vi "CameraSerialController_v04.vi"() -> (4 "图像时间戳":u32=16532020 format="%_32g")   [LabVIEW 2015]
uses:
  <vilib>/Instr/_visa.llb/VISA Configure Serial Port (Instr).vi
  MVCAMSDK.dll
  <vilib>/Analysis/NI_AALBase.lvlib
panel:
  out "连接的字符串":string
  out "转动信号曲线":cluster{"Locations":dbl[], "Amplitudes":dbl[]}[](graph)=[{"Locations"=array[750 elements], "Amplitudes"=array[749 elements]}, {"Locations"=[104.38621227921368, 258.3247060234782, 410.71523318402836, 562.6858730022967, 712.7065754646931], "Amplitudes"=[11153.698204083417, 10559.387052180104, 10974.865031894917, 10500.852817232146, 11059.763900010517]}, {"Locations"=[26.787398227992274, 182.39455189327623, 333.5517219531509, 488.1851999460032, 636.5270621135614], "Amplitudes"=[3284.809720018355, 2039.4564261182056, 3638.2587716464914, 3082.2730888167225, 4217.856016996603]}]
  in  "平移回退":T1=TRUE
  in  "转动回退":T1=TRUE
  in  "转动计数":u16
  in  "转动一次脉冲数":u16=20
  in  "转动前进":T1=TRUE
  in  "平移一次脉冲数":u16=20
  in  "平移计数":u16
  out "variance 2":dbl caption="方差" format="%0.2f"
  in  "flow control (0:none)":u16(ring) caption="流控制（0:无）" items=["无", "XON/XOFF", "RTS/CTS", "XON/XOFF & RTS/CTS", "DTR/DSR", "XON/XOFF & DTR/DSR"]
  in  "stop bits (10: 1 bit)":u16=10 caption="停止位（10: 1位）"
  in  "奇偶 (0:none)":enum16{"None", "Odd", "Even", "Mark", "Space"}(ring) caption="奇偶（0:无）"
  in  "数据比特(默认8)":u16(ring)=8 items=["5"=5, "6"=6, "7"=7, "8"=8]
  in  "波特率(默认9600)":u32=9600
  in  "端口":refnum<visa-resource-name>="COM1"
  in  "平移前进":T1=TRUE
  out "泰伯距离数值":dbl[](array[numeric])=[15.393849374426454, 15.239052716055017, 15.197063981826837, 15.002070246239633]
  out "Locations":dbl[](array[numeric])=[10.438621227921368, 25.832470602347822, 41.07152331840284, 56.268587300229676, 71.27065754646931] caption="上面图像曲线波峰位置"
  out "平移信号曲线":cluster{"Locations":dbl[], "Amplitudes":dbl[]}[](graph)=[{"Locations"=array[750 elements], "Amplitudes"=array[749 elements]}, {"Locations"=[104.38621227921368, 258.3247060234782, 410.71523318402836, 562.6858730022967, 712.7065754646931], "Amplitudes"=[11153.698204083417, 10559.387052180104, 10974.865031894917, 10500.852817232146, 11059.763900010517]}, {"Locations"=[26.787398227992274, 182.39455189327623, 333.5517219531509, 488.1851999460032, 636.5270621135614], "Amplitudes"=[3284.809720018355, 2039.4564261182056, 3638.2587716464914, 3082.2730888167225, 4217.856016996603]}]
  out "光强图 2":dbl[](graph)
  out "variance":dbl caption="方差" format="%0.2f"
  out "相机图像":T2(plugin-control)
  out "横向中心像素光强图":dbl[](graph)
  in  "自定义分辨率设置":bool
  in  "ROI分辨率":T3
  in  "预设分辨率设置":bool
  in  "预设分辨率":T4(radio)
  out "帧速":u32
  out "帧间耗时\n单位：（0.1ms）":u32
  in  "相机枚举":T5(ring)
  in  "自动曝光模式":bool=TRUE caption="软触发"
  in  "手动曝光模式":bool caption="软触发"
  in  "曝光时间，单位微秒":dbl=11000.0 format="%#_6f"
  in  "硬触发模式":bool caption="软触发"
  in  "软触发模式":bool caption="软触发"
  in  "连续模式":bool caption="软触发"
  in  "软触发一帧":bool caption="软触发"
  in  "读取自定义数据":bool
  out "从相机中读出的字符串(32字节)":string
  in  "写入自定义数据":bool
  in  "要写入相机的字符串(32字节)":string
  in  "拍照":bool
  in  "相机参数":bool=TRUE
  in  "Stop":bool
  in  "激活预览":bool=TRUE
  out "Image":T2(plugin-control)
  # "相机原生分辨率设置"
  # "写入自定义数据"
  # "触发设置"
  # "曝光设置"
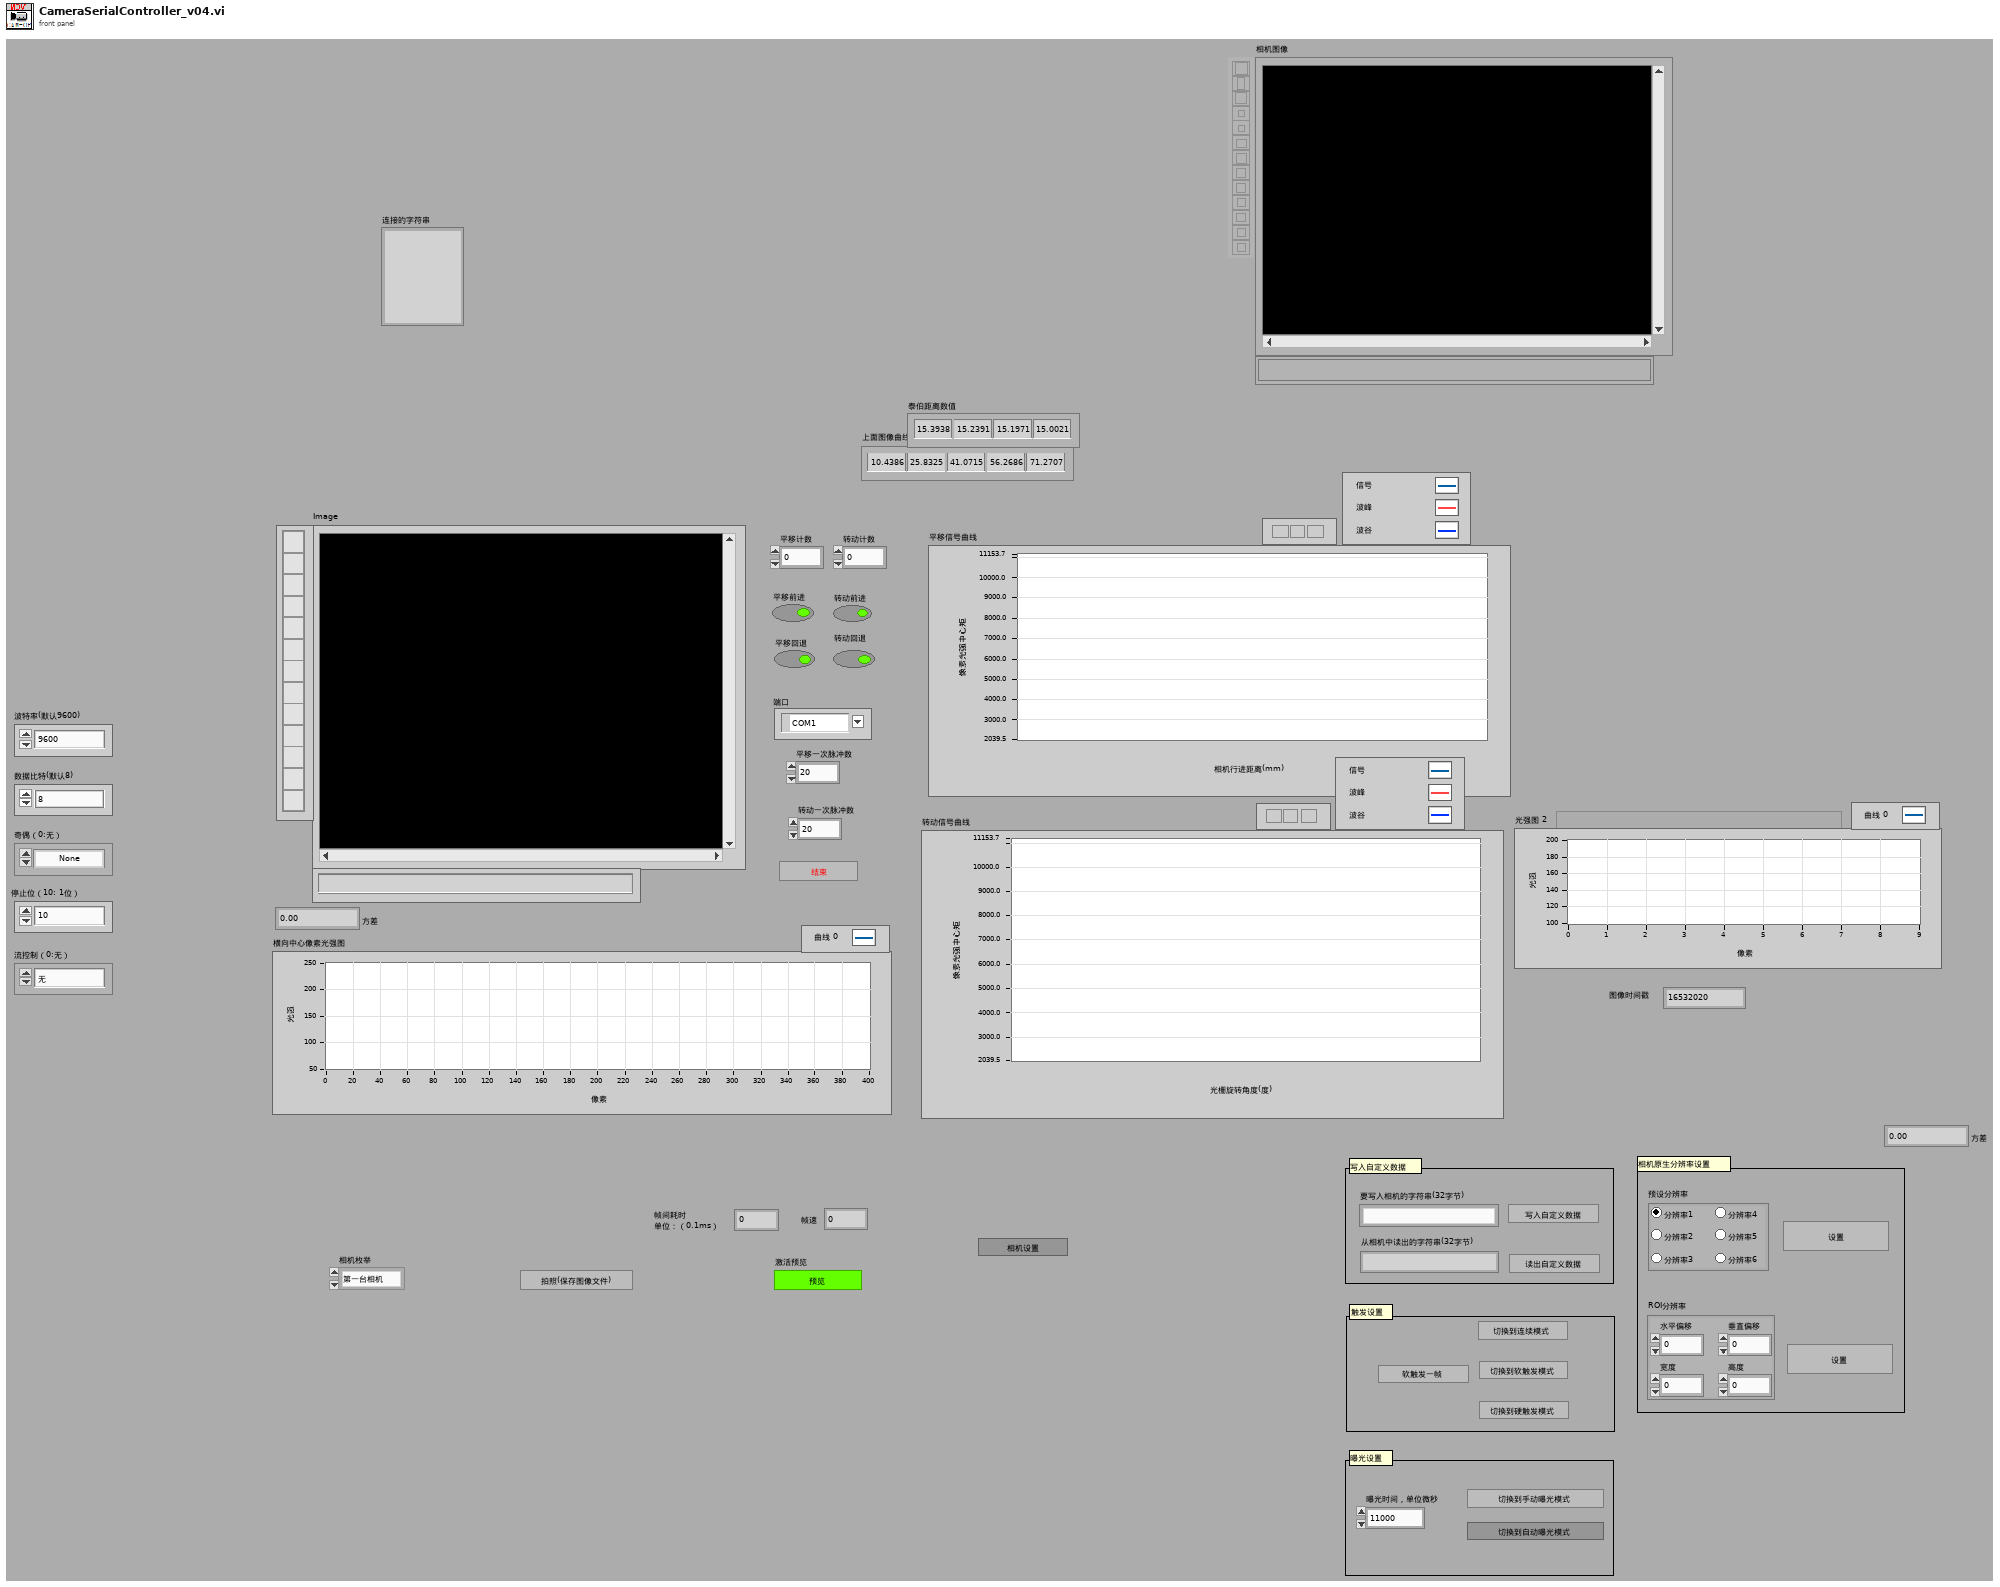
[diagram p1: front panel]
types:
  T1 = typedef "控件 1.ctl" = bool
  T2 = typedef "IMAQ Image.ctl" = refnum<image>
  T3 = cluster{"水平偏移":dbl, "垂直偏移":dbl, "宽度":dbl, "高度":dbl}
  T4 = enum32{"分辨率1", "分辨率2", "分辨率3", "分辨率4", "分辨率5", "分辨率6"}
  T5 = enum16{"第一台相机", "第二台相机", "第三台相机", "第四台相机", "第五台相机"}
  T6 = typedef "Image Type" = u32
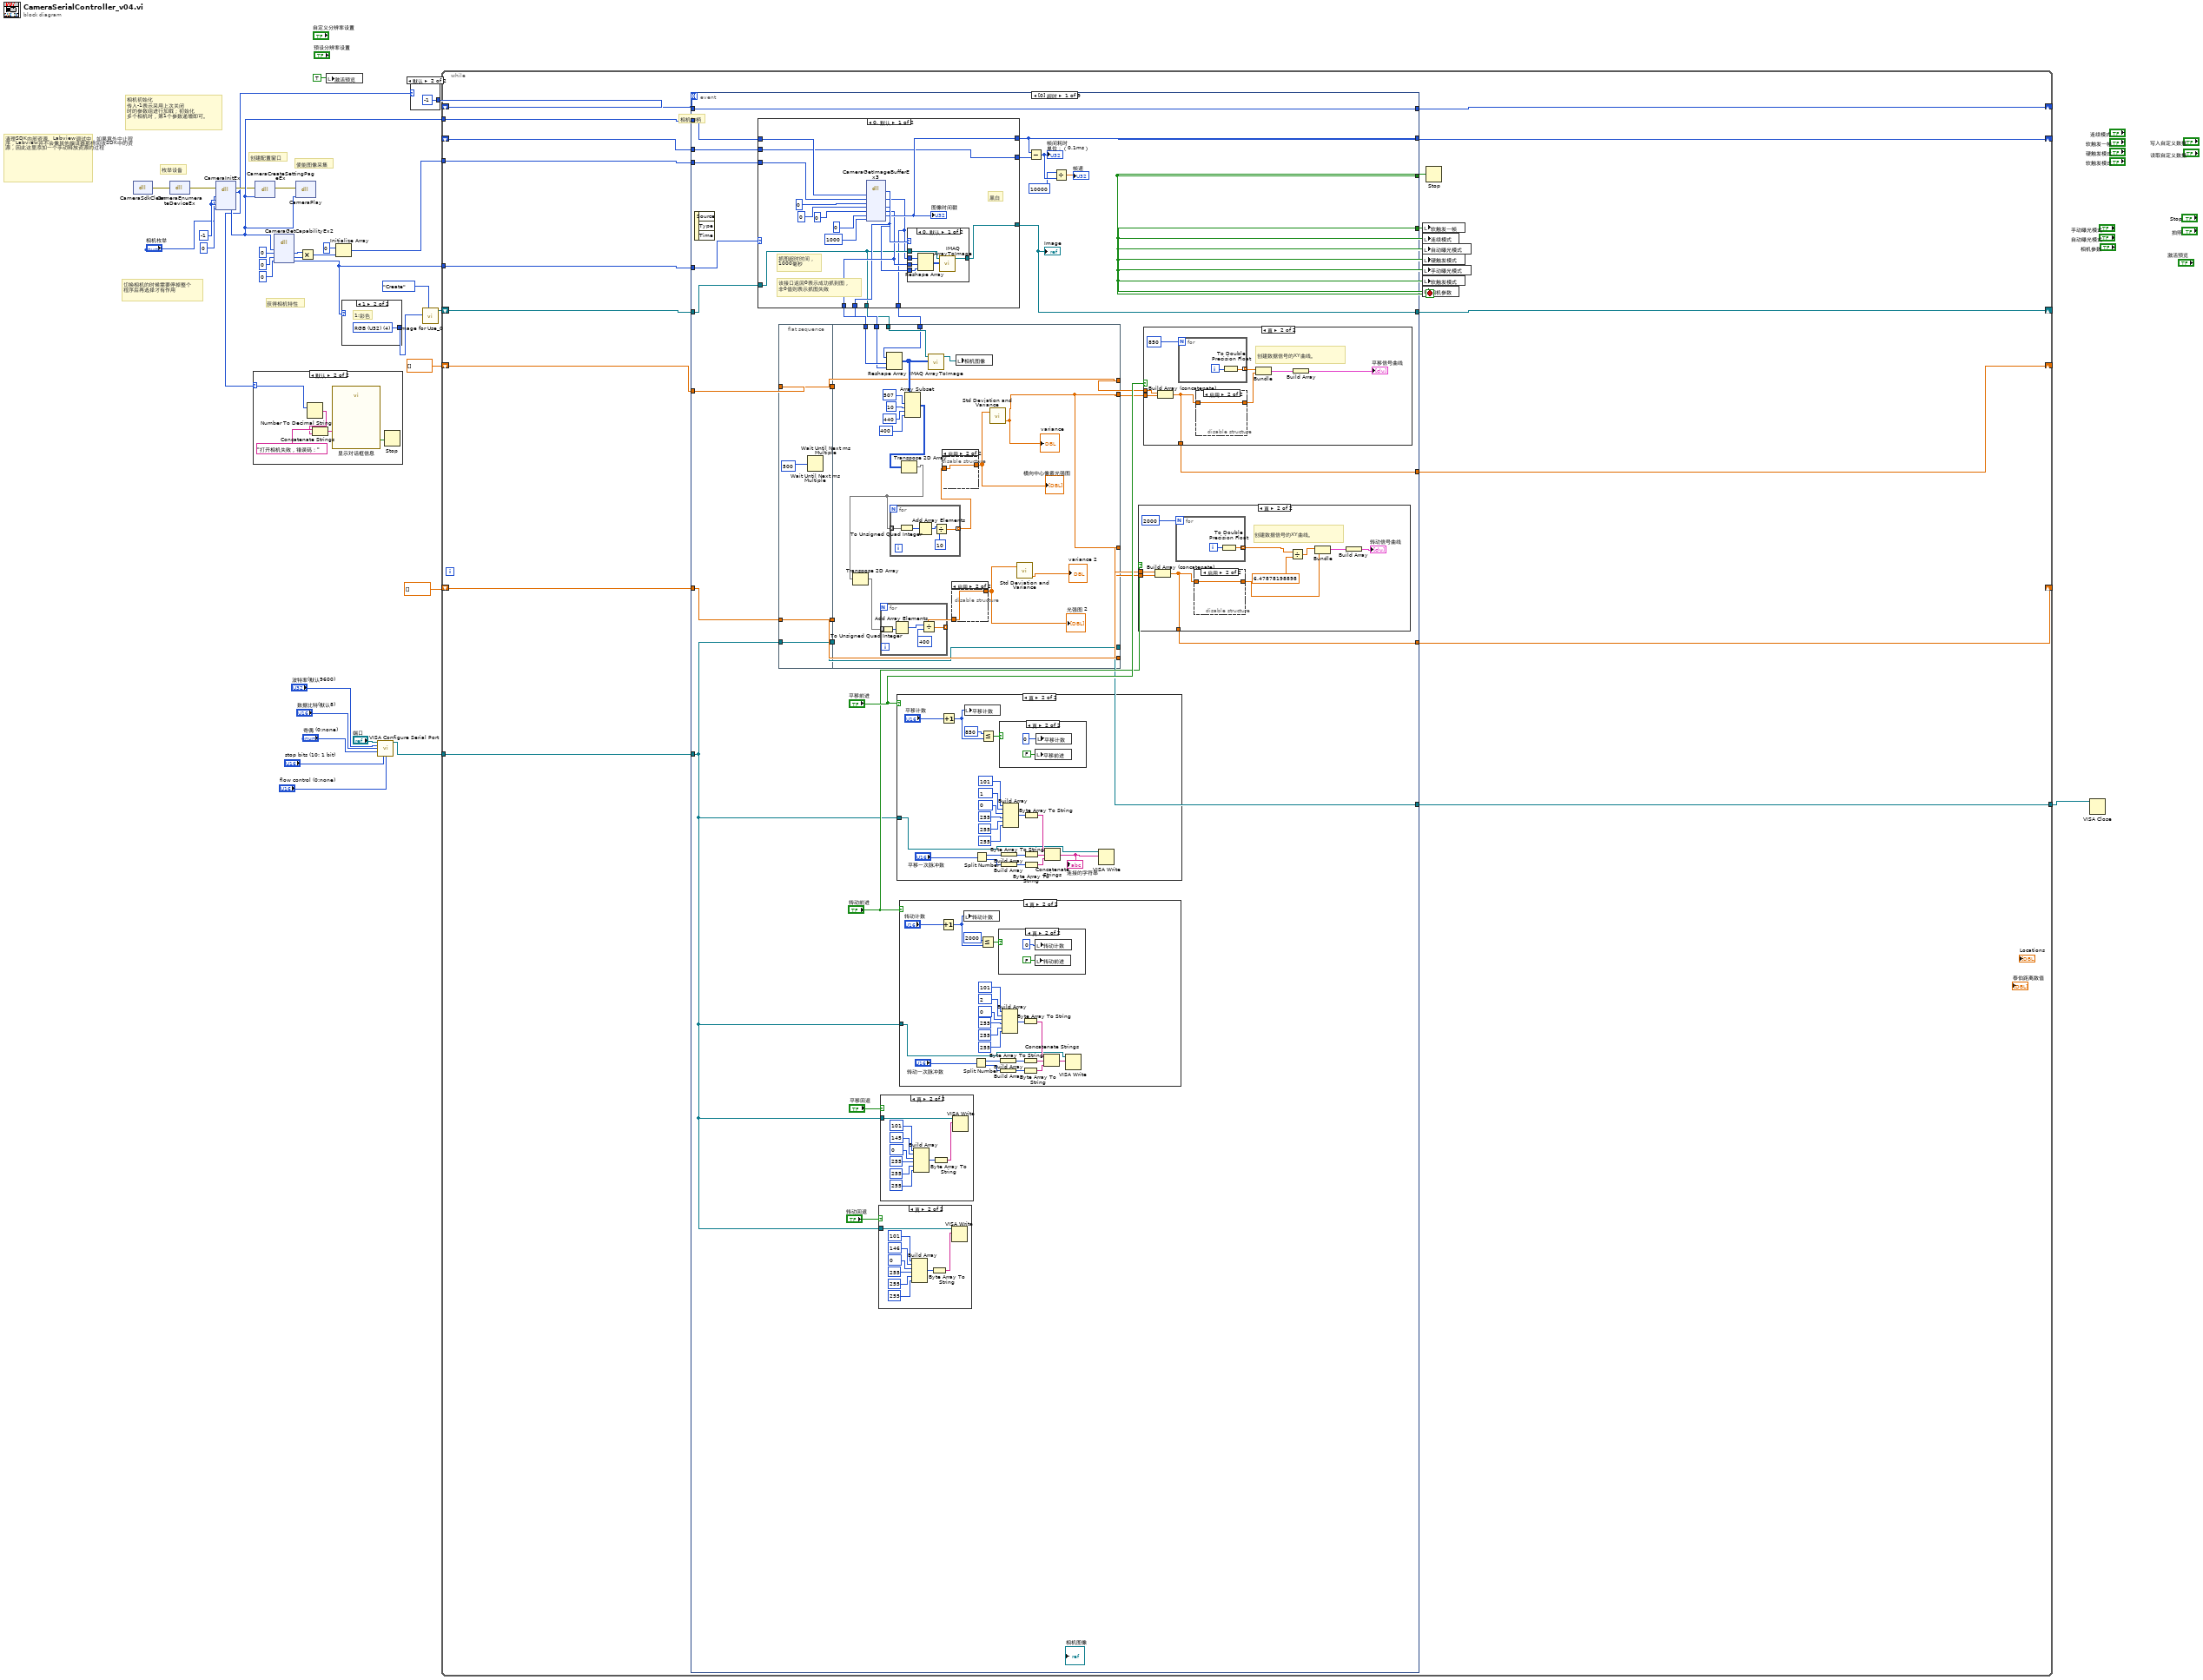
[diagram p0: block diagram]
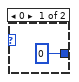
[diagram p2: hidden frame]
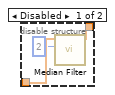
[diagram p4: hidden frame]
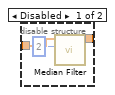
[diagram p5: hidden frame]
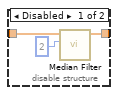
[diagram p7: hidden frame]
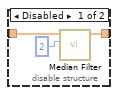
[diagram p9: hidden frame]
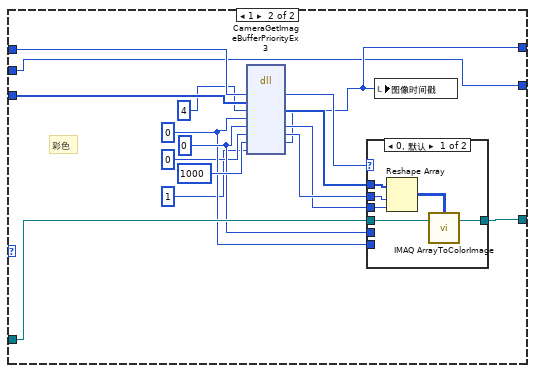
[diagram p17: hidden frame]
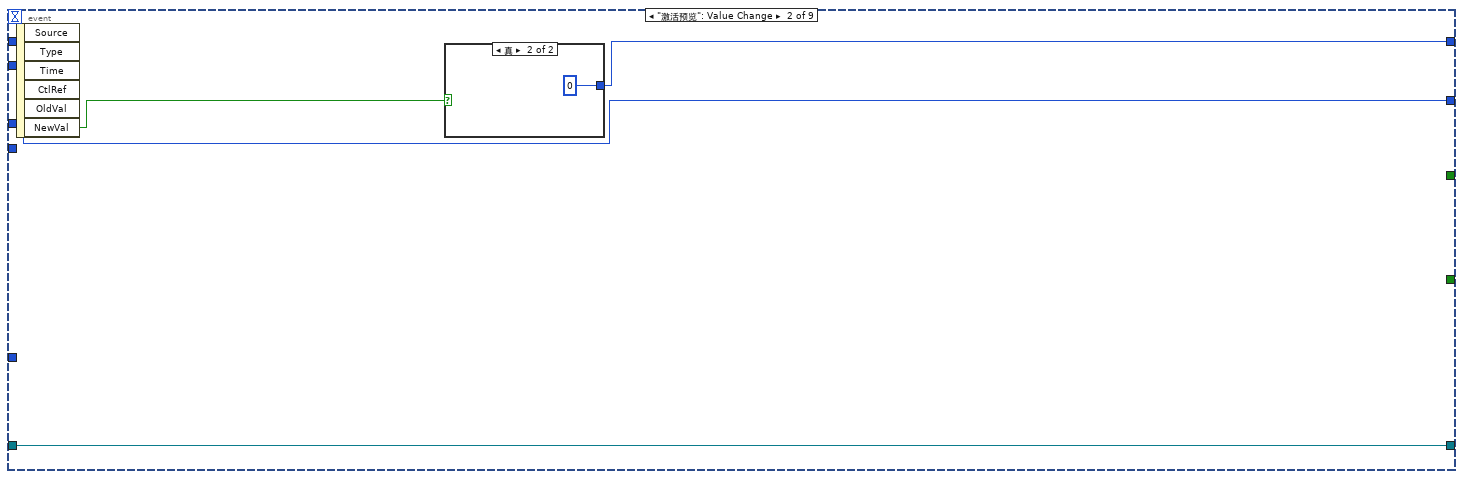
[diagram p19: hidden frame]
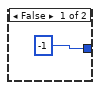
[diagram p20: hidden frame]
diagram:
  w30 = -1
  # "切换相机的时候需要停掉整个\n程序后再选择才有作用"
  # "清理SDK内部资源。Labview调试中，如果意外中止程序，Labview并不会像其他编译器那样回收SDK中的资源，因此这里添加一个手动释放资源的过程"
  # "使能图像采集"
  # "获得相机特性"
  # "创建配置窗口"
  # "相机初始化\n传入-1表示采用上次关闭\n时的参数组进行加载；初始化\n多个相机时，第1个参数递增即可。"
  # "枚举设备"
  n1 = dll-call lib="MVCAMSDK.dll" fn="CameraSdkClean"() -> (error out=w31:errorcluster)  [unwired: 4 in, 1 out]
  n2 = dll-call lib="MVCAMSDK.dll" fn="CameraEnumerateDeviceEx"(error in=w31) -> (error out=w28:errorcluster)  [unwired: 3 in, 1 out]
  n3 = dll-call lib="MVCAMSDK.dll" fn="CameraInitEx"(error in=w28, "相机索引值"="相机枚举", "参数加载方式"=w30, "要加载的参数组索引"=w30, "相机句柄"=0) -> (error out=w17:errorcluster, "返回类型"=w12:i32, "相机句柄"=w19:i32)  [unwired: 5 in, 1 out]
  n4 = case shown="默认" w12 {
    selector: w12 -> [_ w37]
    frame 0 {
    }
    frame Default {
      n5 = Number To Decimal String(number=w37) -> (decimal integer string=w34:string)  [unwired: 1 in]
      n6 = Concatenate Strings("打开相机失败，错误码：" ("字符串"), w34) -> (w36:string)
      n7 = call "显示对话框信息"("Message"=w36) -> ("结束"=w38:bool)  [unwired: 9 in, 1 out]
      n8 = Stop(stop? (T)=w38) -> ()
    }
  }
  n9 = dll-call lib="MVCAMSDK.dll" fn="CameraCreateSettingPageEx"(error in=w17, "相机句柄"=w19) -> (error out=w20:errorcluster)  [unwired: 4 in, 1 out]
  n10 = dll-call lib="MVCAMSDK.dll" fn="CameraGetCapabilityEx2"("相机句柄"=w19, "图像最大宽度"=0, "图像最大高度"=0, "是否是彩色相机(返回0:黑白;1:彩色)"=0) -> ("图像最大宽度"=w22:i32, "图像最大高度"=w21:i32, "是否是彩色相机(返回0:黑白;1:彩色)"=w16:i32)  [unwired: 5 in, 2 out]
  n11 = dll-call lib="MVCAMSDK.dll" fn="CameraPlay"(error in=w20, "相机句柄"=w19) -> ()  [unwired: 4 in, 2 out]
  n12 = Multiply(x=w22, y=w21) -> (x*y=w26:i32)
  n13 = local write "激活预览"(TRUE ("激活预览")) -> ()
  n14 = Initialize Array(0, w26) -> (w18:i32[])
  n15 = case shown="1" w16 {
    tunnel: [_ w39] -> w32
    frame 0, Default {
      # "0:黑白;"
    }
    frame 1 {
      w39 = T6 4 items=["Grayscale (U8)", "Grayscale (I16)", "Grayscale (SGL)", "Complex (CSG)", "RGB (U32)", "HSL (U32)", "RGB (U64)", "Grayscale (U16)"] ("Image Type")
      # "1:彩色"
    }
  }
  n16 = call-poly "VISA Configure Serial Port"("VISA resource name"="端口", "baud rate (9600)"="波特率(默认9600)", "data bits (8)"="数据比特(默认8)", "parity (0:none)"="奇偶 (0:none)", "stop bits (10: 1 bit)"="stop bits (10: 1 bit)", "flow control (0:none)"="flow control (0:none)") -> ("VISA resource name out"=w4:refnum<visa-resource-name>)  [unwired: 8 in, 1 out]
  n17 = case shown="默认" w12 {
    tunnel: [0 -1] -> w11
    frame 0 {
    }
    frame Default {
    }
  }
  n18 = call "Image for Use_0.vi"("Command"=enum16{"Create", "Use", "Copy in", "Dispose"}."Create", "Image Type"=w32) -> ("Image out"=w15:T2)  [unwired: 8 in, 1 out]
  n19 = while {
    tunnel: w19 -> [w55]
    tunnel: w18 -> [w57]
    tunnel: w16 -> [w58]
    shift-right: [w54] -> _
    shift-left: w11 -> [w53]
    shift-right: [w51] -> _
    shift-left: w15 -> [w56]
    shift-right: [w50] -> _
    shift-left: _ -> [w49]
    tunnel: w4 -> [w47]
    tunnel: [w46] -> w3
    shift-right: [w44] -> _
    shift-left: dbl[] [] -> [w45]
    shift-right: [w43] -> _
    shift-left: dbl[] [] -> [w42]
    stop <- w48 stop-if-true
    # "相机句柄"
    n20 = event shown="[0] 超时" {
      selector: _ -> [_ _ _ _ _ _ _ _ _]
      dyn-events: _ -> [_ _ _ _ _ _ _ _ _]
      timeout: w53 -> [_ _ _ _ _ _ _ _ _]
      tunnel: [_ _ _ _ _ _ _ _ TRUE] -> w48
      tunnel: w57 -> [w90 _ _ _ _ _ _ _ _]
      tunnel: w58 -> [w89 _ _ _ _ _ _ _ _]
      tunnel: w55 -> [w91 _ w286 w304 w319 _ w333 w356 w436]
      tunnel: w56 -> [w88 w279 w285 w303 w318 w323 w332 w358 w434]
      tunnel: [w87 w280 w287 w305 w320 w324 w334 w359 w437] -> w54
      tunnel: w53 -> [w87 _ w287 w305 w320 w324 w334 w359 w437]
      tunnel: [_ _ _ _ _ _ _ _ FALSE] -> w52
      tunnel: [w86 w279 w285 w303 w318 w323 w332 w358 w434] -> w51
      tunnel: [w83 w278 w284 w302 w317 w322 w331 w350 w433] -> w50
      tunnel: w49 -> [w85 w278 w284 w302 w317 w322 w331 w350 w433]
      tunnel: w47 -> [w62 _ _ _ _ _ _ _ _]
      tunnel: [w61 _ _ _ _ _ _ _ _] -> w46
      tunnel: w45 -> [w69 _ _ _ _ _ _ _ _]
      tunnel: [w72 _ _ _ _ _ _ _ _] -> w44
      tunnel: [w71 _ _ _ _ _ _ _ _] -> w43
      tunnel: w42 -> [w64 _ _ _ _ _ _ _ _]
      event Timeout {
        n21 = event-data() -> ()  [unwired: 1 in, 3 out]
        n22 = case shown="0, 默认" w89 {
          tunnel: w90 -> [w247 w270]
          tunnel: w88 -> [w234 w269]
          tunnel: w91 -> [w239 w268]
          tunnel: [w240 w258] -> w86
          tunnel: [w238 w257] -> w83
          tunnel: w85 -> [w237 w256]
          tunnel: [w237 w256] -> w84
          tunnel: [w236 _] -> w79
          tunnel: [w235 _] -> w78
          tunnel: [w234 _] -> w77
          tunnel: [w233 _] -> w76
          frame 0, Default {
            # "黑白"
            # "该接口返回0表示成功抓到图，\n非0值则表示抓图失败"
            # "抓图超时时间，\n1000毫秒"
            n23 = dll-call lib="MVCAMSDK.dll" fn="CameraGetImageBufferEx3"("相机句柄"=w239, "图像数据缓冲区"=w247, "图像输出格式(0:8位灰度;1:24位彩色;2:32位彩色，3：BGR24彩色 4：BGRA32位彩色)"=0, "图像宽度"=0, "图像高度"=0, "时间戳(单位为100微秒)"=0, "抓图超时时间(毫秒)"=1000) -> ("返回类型"=w242:i32, "图像数据缓冲区"=w233:u8[], "图像宽度"=w235:i32, "图像高度"=w236:i32, "时间戳(单位为100微秒)"=w238:u32)  [unwired: 6 in, 2 out]
            "图像时间戳" <- w238
            n24 = case shown="0, 默认" w242 {
              tunnel: w233 -> [w253 _]
              tunnel: w234 -> [w250 w254]
              tunnel: w236 -> [w252 _]
              tunnel: w235 -> [w251 _]
              tunnel: [w248 w254] -> w240
              frame 0, Default {
                n25 = Reshape Array(w253, w252, w251) -> (w249:u8[][])
                n26 = call "IMAQ ArrayToImage"("Image Pixels (U8)"=w249, "Image"=w250) -> ("Image Out"=w248:T2)  [unwired: 8 in, 1 out]
              }
              frame -12 {
              }
            }
          }
          frame 1 {
            w260 = 0
            w261 = 0
            # "彩色"
            n27 = dll-call lib="MVCAMSDK.dll" fn="CameraGetImageBufferPriorityEx3"("相机句柄"=w268, "图像数据缓冲区"=w270, "图像输出格式(0:8位灰度;1:24位彩色;2:32位彩色)"=4, "图像宽度"=w260, "图像高度"=w261, "时间戳（单位为100微秒）"=0, "抓图超时时间(毫秒)"=1000, "取图优先级(0: 取最旧   1:取最新)"=1) -> ("返回类型"=w262:i32, "图像数据缓冲区"=w265:u32[], "图像宽度"=w263:i32, "图像高度"=w264:i32, "时间戳（单位为100微秒）"=w257:u32)  [unwired: 7 in, 2 out]
            n28 = case shown="0, 默认" w262 {
              tunnel: w265 -> [w275 _]
              tunnel: w269 -> [w274 w277]
              tunnel: w264 -> [w273 _]
              tunnel: w263 -> [w272 _]
              tunnel: w261 -> [_ _]
              tunnel: w260 -> [_ _]
              tunnel: [w271 w277] -> w258
              frame 0, Default {
                n29 = Reshape Array(w275, w273, w272) -> (w276:u32[][])
                n30 = call "IMAQ ArrayToColorImage"("Image Pixels (U32)"=w276, "Image"=w274) -> ("Image Out"=w271:T2)  [unwired: 3 in, 1 out]
              }
              frame -12 {
              }
            }
            n31 = local write "图像时间戳"(w257) -> ()
          }
        }
        "Image" <- w86
        n32 = flat-sequence {
          tunnel: w69 -> [w96]
          tunnel: [w96] -> w67
          tunnel: [w93] -> w65
          tunnel: w64 -> [w93]
          tunnel: [w92] -> w63
          tunnel: w62 -> [w92]
          tunnel: w79 -> [w117]
          tunnel: w78 -> [w116]
          tunnel: w77 -> [w115]
          tunnel: w76 -> [w114]
          tunnel: [w99] -> w59
          tunnel: [w103] -> w68
          tunnel: w67 -> [w103]
          tunnel: [w102] -> w66
          tunnel: w65 -> [w102]
          tunnel: [w101] -> w61
          tunnel: w63 -> [w101]
          tunnel: [w99] -> w60
          frame #0 {
            n33 = Wait Until Next ms Multiple(millisecond multiple=u32 500 ("毫秒倍数")) -> ()  [unwired: 1 out]
            n34 = Wait Until Next ms Multiple(millisecond multiple=u32 500 ("毫秒倍数")) -> ()  [unwired: 1 out]
          }
          frame #1 {
            n35 = Reshape Array(w114, w117, w116) -> (w113:u8[][])
            n36 = Array Subset(array=w113, index (row)=507 ("索引"), length (row)=10 ("长度"), index (col)=440 ("长度"), length (col)=400 ("索引")) -> (w97:u8[][])
            n37 = Transpose 2D Array(2D array=w97) -> (transposed array=w98:u8[][])
            n38 = Transpose 2D Array(2D array=w98) -> (transposed array=w110:u8[][])
            n39 = for {
              tunnel: w110 -> [w122] mode=indexing
              tunnel: [w120] -> w111 mode=indexing
              n40 = To Unsigned Quad Integer(1:w122) -> (0:w121:u64[])
              n41 = Add Array Elements(numeric array=w121) -> (sum=w123:u64)
              n42 = Divide(x=w123, y=u64 400) -> (x/y=w120:dbl)
            }
            n43 = for {
              tunnel: w98 -> [w131] mode=indexing
              tunnel: [w129] -> w112 mode=indexing
              n44 = To Unsigned Quad Integer(1:w131) -> (0:w130:u64[])
              n45 = Add Array Elements(numeric array=w130) -> (sum=w132:u64)
              n46 = Divide(x=w132, y=u64 10) -> (x/y=w129:dbl)
            }
            n47 = call "IMAQ ArrayToImage"("Image Pixels (U8)"=w113, "Image"=w115) -> ("Image Out"=w118:T2)  [unwired: 8 in, 1 out]
            n48 = disable-structure shown="启用" {
              disable-tunnel: w112 -> [w135 w136]
              disable-tunnel: [w133 w136] -> w109
              frame Disabled {
                n49 = call <vilib>:"Median Filter.vi"("left rank"=2, "X"=w135) -> ("Filtered X"=w133:dbl[])  [unwired: 8 in, 1 out]
              }
              frame Enabled {
              }
            }
            "横向中心像素光强图" <- w109
            n50 = disable-structure shown="启用" {
              disable-tunnel: w111 -> [w126 w127]
              disable-tunnel: [w124 w127] -> w108
              frame Disabled {
                n51 = call <vilib>:"Median Filter.vi"("left rank"=2, "X"=w126) -> ("Filtered X"=w124:dbl[])  [unwired: 8 in, 1 out]
              }
              frame Enabled {
              }
            }
            "光强图 2" <- w108
            n52 = local write "相机图像"(w118) -> ()
            n53 = call <vilib>:"Std Deviation and Variance.vi"("X"=w109) -> ("variance"=w99:dbl)  [unwired: 1 in, 2 out]
            "variance" <- w99
            n54 = call <vilib>:"Std Deviation and Variance.vi"("X"=w108) -> ("variance"=→"variance 2":dbl)  [unwired: 1 in, 2 out]
          }
        }
        n55 = case shown="真" "转动回退" {
          tunnel: w62 -> [_ w170]
          frame False {
          }
          frame True {
            n56 = Build Array(101, 146, 0, 255, 255, 255) -> (w171:i32[])
            n57 = Byte Array To String(unsigned byte array=w171) -> (string=w169:string)
            n58 = VISA Write(VISA resource name=w170, write buffer=w169) -> ()  [unwired: 1 in, 3 out]
          }
        }
        n59 = case shown="真" "平移回退" {
          tunnel: w62 -> [_ w179]
          frame False {
          }
          frame True {
            n60 = Build Array(101, 145, 0, 255, 255, 255) -> (w180:i32[])
            n61 = Byte Array To String(unsigned byte array=w180) -> (string=w178:string)
            n62 = VISA Write(VISA resource name=w179, write buffer=w178) -> ()  [unwired: 1 in, 3 out]
          }
        }
        n63 = case shown="真" "平移前进" {
          tunnel: w62 -> [_ w213]
          frame False {
          }
          frame True {
            n64 = Increment(x="平移计数") -> (x+1=w211:u16)
            n65 = local write "平移计数"(w211) -> ()
            n66 = Split Number(x="平移一次脉冲数") -> (hi(x)=w221:u8, lo(x)=w220:u8)
            n67 = Less Or Equal?(x=850, y=w211) -> (x <= y?=w223:bool)
            n68 = case shown="真" w223 {
              frame False {
              }
              frame True {
                n69 = local write "平移前进"(T1 FALSE ("平移前进")) -> ()
                n70 = local write "平移计数"(u16 0 ("平移计数 2")) -> ()
              }
            }
            n71 = Build Array(w221) -> (w219:u8[])
            n72 = Build Array(w220) -> (w218:u8[])
            n73 = Build Array(101, 1, 0, 255, 255, 255) -> (w217:i32[])
            n74 = Byte Array To String(unsigned byte array=w217) -> (string=w216:string)
            n75 = Byte Array To String(unsigned byte array=w219) -> (string=w215:string)
            n76 = Byte Array To String(unsigned byte array=w218) -> (string=w214:string)
            n77 = Concatenate Strings(w216, w215, w214) -> (w210:string)
            "连接的字符串" <- w210
            n78 = VISA Write(VISA resource name=w213, write buffer=w210) -> ()  [unwired: 1 in, 3 out]
          }
        }
        n79 = case shown="真" "转动前进" {
          tunnel: w62 -> [_ w191]
          frame False {
          }
          frame True {
            n80 = Increment(x="转动计数") -> (x+1=w189:u16)
            n81 = local write "转动计数"(w189) -> ()
            n82 = Split Number(x="转动一次脉冲数") -> (hi(x)=w199:u8, lo(x)=w198:u8)
            n83 = Less Or Equal?(x=2000, y=w189) -> (x <= y?=w201:bool)
            n84 = case shown="真" w201 {
              frame False {
              }
              frame True {
                n85 = local write "转动前进"(T1 FALSE ("平移前进")) -> ()
                n86 = local write "转动计数"(u16 0 ("平移计数")) -> ()
              }
            }
            n87 = Build Array(w199) -> (w197:u8[])
            n88 = Build Array(w198) -> (w196:u8[])
            n89 = Build Array(101, 2, 0, 255, 255, 255) -> (w195:i32[])
            n90 = Byte Array To String(unsigned byte array=w195) -> (string=w194:string)
            n91 = Byte Array To String(unsigned byte array=w197) -> (string=w193:string)
            n92 = Byte Array To String(unsigned byte array=w196) -> (string=w192:string)
            n93 = Concatenate Strings(w194, w193, w192) -> (w188:string)
            n94 = VISA Write(VISA resource name=w191, write buffer=w188) -> ()  [unwired: 1 in, 3 out]
          }
        }
        n95 = Subtract(x=w83, y=w84) -> (x-y=w82:u32)
        "帧间耗时\n单位：（0.1ms）" <- w82
        n96 = Divide(x=u32 10000 ("帧间耗时"), y=w82) -> (x/y=→"帧速":dbl)
        n97 = case shown="真" "转动前进" {
          tunnel: w60 -> [_ w143]
          tunnel: w66 -> [w137 w142]
          tunnel: [w137 w141] -> w71
          frame False {
          }
          frame True {
            # "创建数据信号的XY曲线。"
            n98 = Build Array (concatenate)(w142, w143) -> (w141:dbl[])
            n99 = for {
              N: i64 2000 ("数值") -> [_]
              tunnel: [w148] -> w140 mode=indexing
              i -> [w149]
              n100 = To Double Precision Float(number=w149) -> (double precision float=w148:dbl)
            }
            n101 = disable-structure shown="启用" {
              disable-tunnel: w141 -> [w151 w153]
              disable-tunnel: [w150 w153] -> w145
              frame Disabled {
                n102 = call <vilib>:"Median Filter.vi"("left rank"=2, "X"=w151) -> ("Filtered X"=w150:dbl[])  [unwired: 8 in, 1 out]
              }
              frame Enabled {
              }
            }
            n103 = Divide(x=w140, y=6.47878198898) -> (x/y=w138:dbl[])
            n104 = Bundle(w138, w145) -> (w147:cluster{dbl[], dbl[]})  [unwired: 1 in]
            n105 = Build Array(w147) -> (→"转动信号曲线":cluster{dbl[], dbl[]}[])
          }
        }
        n106 = case shown="真" "平移前进" {
          tunnel: w68 -> [w154 w156]
          tunnel: w59 -> [_ w157]
          tunnel: [w154 w155] -> w72
          frame False {
          }
          frame True {
            # "创建数据信号的XY曲线。"
            n107 = Build Array (concatenate)(w156, w157) -> (w155:dbl[])
            n108 = for {
              N: i64 850 ("数值") -> [_]
              tunnel: [w163] -> w161 mode=indexing
              i -> [w164]
              n109 = To Double Precision Float(number=w164) -> (double precision float=w163:dbl)
            }
            n110 = disable-structure shown="启用" {
              disable-tunnel: w155 -> [w166 w168]
              disable-tunnel: [w165 w168] -> w160
              frame Disabled {
                n111 = call <vilib>:"Median Filter.vi"("left rank"=2, "X"=w166) -> ("Filtered X"=w165:dbl[])  [unwired: 8 in, 1 out]
              }
              frame Enabled {
              }
            }
            n112 = Bundle(w161, w160) -> (w158:cluster{dbl[], dbl[]})  [unwired: 1 in]
            n113 = Build Array(w158) -> (→"平移信号曲线":cluster{dbl[], dbl[]}[])
          }
        }
      }
      event "激活预览": Value Change {
        n114 = event-data() -> ("NewVal"=w281:bool)  [unwired: 1 in, 5 out]
        n115 = case shown="真" w281 {
          tunnel: [-1 0] -> w280
          frame False {
          }
          frame True {
          }
        }
      }
      event "连续模式", "软触发一帧", "硬触发模式", "软触发模式": Value Change {
        n116 = event-data() -> ("CtlRef"=w289:refnum<vi>)  [unwired: 1 in, 5 out]
        n117 = control-ref of="连续模式"() -> (w291:refnum<vi>)
        n118 = control-ref of="硬触发模式"() -> (w292:refnum<vi>)
        n119 = control-ref of="软触发模式"() -> (w293:refnum<vi>)
        n120 = control-ref of="软触发一帧"() -> (w294:refnum<vi>)
        n121 = Build Array ("创建数组")(w291, w292, w293, w294) -> (w290:refnum<vi>[])
        n122 = Search 1D Array(1D array=w290, element=w289) -> (index of element=w288:i32)  [unwired: 1 in]
        n123 = case shown="1" w288 {
          tunnel: w286 -> [w295 w297 w299 w301]
          frame 0, Default {
            # "连续模式"
            n124 = dll-call lib="MVCAMSDK.dll" fn="CameraSetTriggerMode"("相机句柄"=w295, "模式"=0) -> ()  [unwired: 6 in, 2 out]
          }
          frame 1 {
            # "硬触发模式"
            n125 = dll-call lib="MVCAMSDK.dll" fn="CameraSetTriggerMode"("相机句柄"=w297, "模式"=2) -> ()  [unwired: 6 in, 2 out]
          }
          frame 2 {
            # "软触发模式"
            n126 = dll-call lib="MVCAMSDK.dll" fn="CameraSetTriggerMode"("相机句柄"=w299, "模式"=1) -> ()  [unwired: 6 in, 2 out]
          }
          frame 3 {
            # "软触发一帧"
            n127 = dll-call lib="MVCAMSDK.dll" fn="CameraSoftTrigger"("相机句柄"=w301) -> ()  [unwired: 5 in, 2 out]
          }
        }
      }
      event "手动曝光模式", "自动曝光模式": Value Change {
        n128 = event-data() -> ("CtlRef"=w308:refnum<vi>)  [unwired: 1 in, 5 out]
        n129 = control-ref of="自动曝光模式"() -> (w306:refnum<vi>)
        n130 = control-ref of="手动曝光模式"() -> (w309:refnum<vi>)
        n131 = Build Array ("创建数组")(w309, w306) -> (w310:refnum<vi>[])
        n132 = Search 1D Array(1D array=w310, element=w308) -> (index of element=w307:i32)  [unwired: 1 in]
        n133 = case shown="0, 默认" w307 {
          tunnel: w304 -> [w311 w315]
          frame 0, Default {
            # "手动曝光模式"
            n134 = dll-call lib="MVCAMSDK.dll" fn="CameraSetAeState"("相机句柄"=w311, "曝光模式(0手动，1自动)"=0) -> (error out=w314:errorcluster)  [unwired: 6 in, 1 out]
            n135 = dll-call lib="MVCAMSDK.dll" fn="CameraSetExposureTime"(error in=w314, "相机句柄"=w311, "曝光时间，单位微秒"="曝光时间，单位微秒") -> ()  [unwired: 5 in, 2 out]
          }
          frame 1 {
            # "自动曝光模式"
            n136 = dll-call lib="MVCAMSDK.dll" fn="CameraSetAeState"("相机句柄"=w315, "曝光模式(0手动，1自动)"=1) -> ()  [unwired: 6 in, 2 out]
          }
        }
      }
      event "相机参数": Value Change {
        n137 = event-data() -> ()  [unwired: 1 in, 6 out]
        n138 = dll-call lib="MVCAMSDK.dll" fn="CameraShowSettingPage"("相机句柄"=w319, "状态"=TRUE) -> ()  [unwired: 6 in, 2 out]
      }
      event "拍照": Value Change {
        n139 = event-data() -> ()  [unwired: 1 in, 6 out]
        n140 = local read "Image"() -> (w325:T2)
        n141 = Format Date/Time String(time format string (%c)="%Y-%m-%d %H：%M：%S.bmp ") -> (date/time string=w329:string)  [unwired: 2 in]
        n142 = Concatenate Strings("c:\\", w329) -> (w326:string)
        n143 = String To Path(string=w326) -> (path=w328:path)
        n144 = call-poly "IMAQ Write File 2"("File Path"=w328, "Image"=w325) -> ()  [unwired: 8 in, 2 out]
      }
      event "写入自定义数据", "读取自定义数据": Value Change {
        n145 = event-data() -> ("CtlRef"=w336:refnum<vi>)  [unwired: 1 in, 5 out]
        n146 = control-ref of="读取自定义数据"() -> (w338:refnum<vi>)
        n147 = control-ref of="写入自定义数据"() -> (w337:refnum<vi>)
        n148 = Build Array ("创建数组")(w338, w337) -> (w339:refnum<vi>[])
        n149 = Search 1D Array(1D array=w339, element=w336) -> (index of element=w335:i32)  [unwired: 1 in]
        n150 = case shown="0, 默认" w335 {
          tunnel: w333 -> [w340 w347]
          frame 0, Default {
            n151 = Initialize Array(0, 32) -> (w344:i32[])
            n152 = dll-call lib="MVCAMSDK.dll" fn="CameraReadSN"("相机句柄"=w340, "序列号"=w344, "序列号级别，[0,1,2],0级为只读，1,2级可写"=1) -> ("序列号"=w342:u8[])  [unwired: 6 in, 2 out]
            n153 = Byte Array To String(unsigned byte array=w342) -> (string=→"从相机中读出的字符串(32字节)":string)
          }
          frame 1 {
            n154 = dll-call lib="MVCAMSDK.dll" fn="CameraWriteSN"("相机句柄"=w347, "序列号(固定为32个字节)"="要写入相机的字符串(32字节)", "序列号级别，[0,1,2]对应3级序列号，其中0级为只读，1,2级可写"=1) -> ()  [unwired: 7 in, 2 out]
          }
        }
      }
      event "预设分辨率设置", "自定义分辨率设置": Value Change {
        n155 = event-data() -> ("CtlRef"=w352:refnum<vi>)  [unwired: 1 in, 5 out]
        n156 = control-ref of="预设分辨率设置"() -> (w354:refnum<vi>)
        n157 = control-ref of="自定义分辨率设置"() -> (w353:refnum<vi>)
        n158 = Build Array ("创建数组")(w354, w353) -> (w355:refnum<vi>[])
        n159 = Search 1D Array(1D array=w355, element=w352) -> (index of element=w351:i32)  [unwired: 1 in]
        n160 = case shown="1" w351 {
          tunnel: "预设分辨率" -> [w361 _]
          tunnel: w356 -> [w360 w422]
          frame 0, Default {
            n161 = case shown="\"分辨率2\"" w361 {
              tunnel: w360 -> [w362 w381 w382 w392 w402 w412]
              frame "分辨率1", Default {
                n162 = dll-call lib="MVCAMSDK.dll" fn="CameraSetImageResolutionEx"("相机句柄"=w362, "预设分辨率索引"=0, "Mode"=0, "ModeSize"=u32 0, "x"=0, "y"=u32 0 ("ModeSize"), "width"=0, "height"=0, "ZoomWidth"=0, "ZoomHeight"=0) -> ()  [unwired: 14 in, 2 out]
              }
              frame "分辨率2" {
                n163 = dll-call lib="MVCAMSDK.dll" fn="CameraSetImageResolutionEx"("相机句柄"=w381, "预设分辨率索引"=1, "Mode"=0, "ModeSize"=u32 0, "x"=0, "y"=u32 0 ("ModeSize"), "width"=0, "height"=0, "ZoomWidth"=0, "ZoomHeight"=0) -> ()  [unwired: 14 in, 2 out]
              }
              frame "分辨率3" {
                n164 = dll-call lib="MVCAMSDK.dll" fn="CameraSetImageResolutionEx"("相机句柄"=w382, "预设分辨率索引"=2, "Mode"=0, "ModeSize"=u32 0, "x"=0, "y"=u32 0 ("ModeSize"), "width"=0, "height"=0, "ZoomWidth"=0, "ZoomHeight"=0) -> ()  [unwired: 14 in, 2 out]
              }
              frame "分辨率4" {
                n165 = dll-call lib="MVCAMSDK.dll" fn="CameraSetImageResolutionEx"("相机句柄"=w392, "预设分辨率索引"=3, "Mode"=0, "ModeSize"=u32 0, "x"=0, "y"=u32 0 ("ModeSize"), "width"=0, "height"=0, "ZoomWidth"=0, "ZoomHeight"=0) -> ()  [unwired: 14 in, 2 out]
              }
              frame "分辨率5" {
                n166 = dll-call lib="MVCAMSDK.dll" fn="CameraSetImageResolutionEx"("相机句柄"=w402, "预设分辨率索引"=4, "Mode"=0, "ModeSize"=u32 0, "x"=0, "y"=u32 0 ("ModeSize"), "width"=0, "height"=0, "ZoomWidth"=0, "ZoomHeight"=0) -> ()  [unwired: 14 in, 2 out]
              }
              frame "分辨率6" {
                n167 = dll-call lib="MVCAMSDK.dll" fn="CameraSetImageResolutionEx"("相机句柄"=w412, "预设分辨率索引"=5, "Mode"=0, "ModeSize"=u32 0, "x"=0, "y"=u32 0 ("ModeSize"), "width"=0, "height"=0, "ZoomWidth"=0, "ZoomHeight"=0) -> ()  [unwired: 14 in, 2 out]
              }
            }
          }
          frame 1 {
            n168 = Unbundle("ROI分辨率") -> ("水平偏移"=w424:dbl, "垂直偏移"=w425:dbl, "宽度"=w426:dbl, "高度"=w427:dbl)
            n169 = dll-call lib="MVCAMSDK.dll" fn="CameraSetImageResolutionEx"("相机句柄"=w422, "预设分辨率索引"=255, "Mode"=0, "ModeSize"=u32 0, "x"=w424, "y"=w425, "width"=w426, "height"=w427, "ZoomWidth"=0, "ZoomHeight"=u32 0 ("ModeSize")) -> ()  [unwired: 14 in, 2 out]
          }
        }
      }
      event "Stop": Value Change {
        # "反初始化相机"
        n170 = event-data() -> ()  [unwired: 1 in, 6 out]
        n171 = dll-call lib="MVCAMSDK.dll" fn="CameraUnInit"("相机句柄"=w436) -> ()  [unwired: 5 in, 2 out]
      }
    }
    n172 = local write "软触发一帧"(w52) -> ()
    n173 = local write "连续模式"(w52) -> ()
    n174 = local write "自动曝光模式"(w52) -> ()
    n175 = local write "硬触发模式"(w52) -> ()
    n176 = local write "手动曝光模式"(w52) -> ()
    n177 = local write "软触发模式"(w52) -> ()
    n178 = local write "相机参数"(w52) -> ()
    n179 = Stop(stop? (T)=w48) -> ()
  }
  n180 = VISA Close(VISA resource name=w3) -> ()  [unwired: 1 in, 1 out]
